vi "Convert Measurement Units.vi"(8 "error in (no error)":errorcluster, 9 "Units (0:Hz)":u16(ring) items=["Hz", "KHz", "MHz", "GHz"], 10 "Measurement Value (0)":dbl, 11 "VISA resource name":refnum<visa-resource-name>) -> (0 "error out":errorcluster, 2 "Final Value":dbl, 3 "VISA resource name out":refnum<visa-resource-name>)   [LabVIEW 2016, in "Tektronix DPO MSO 2000 4000 Series.lvlib"]
doc: "Converts measurement units from kHz, MHz and GHz to their appropriate representation in Hz."
uses:
  Tektronix DPO MSO 2000 4000 Series.lvlib
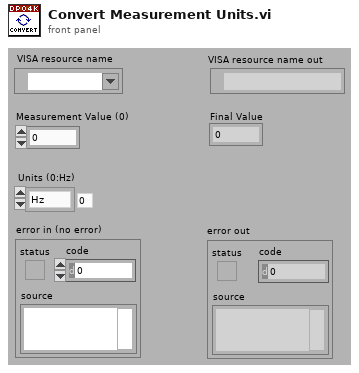
[diagram p1: front panel]
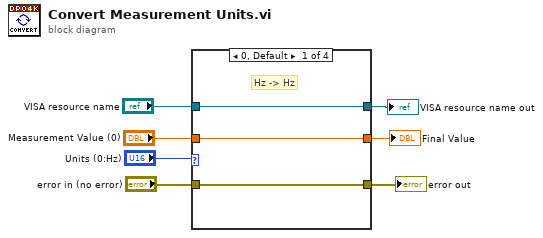
[diagram p0: block diagram]
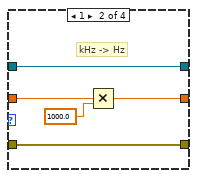
[diagram p2: hidden frame]
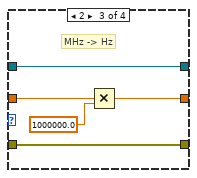
[diagram p3: hidden frame]
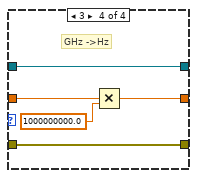
[diagram p4: hidden frame]
diagram:
  n1 = case shown="0, Default" "Units (0:Hz)" {
    tunnel: "Measurement Value (0)" -> [w8 w13 w17 w21]
    tunnel: "VISA resource name" -> [w10 w15 w20 w25]
    tunnel: [w10 w15 w20 w25] -> w2
    tunnel: "error in (no error)" -> [w9 w14 w19 w24]
    tunnel: [w9 w14 w19 w24] -> w3
    tunnel: [w8 w11 w16 w22] -> w1
    frame 0, Default {
      # "Hz -> Hz"
    }
    frame 1 {
      # "kHz -> Hz"
      n2 = Multiply(x=w13, y=1000.0) -> (x*y=w11:dbl)
    }
    frame 2 {
      # "MHz -> Hz"
      n3 = Multiply(x=w17, y=1000000.0) -> (x*y=w16:dbl)
    }
    frame 3 {
      # "GHz ->Hz"
      n4 = Multiply(x=w21, y=1000000000.0) -> (x*y=w22:dbl)
    }
  }
  "error out" <- w3
  "VISA resource name out" <- w2
  "Final Value" <- w1
